vi "Example Callback - EdgeCount Callback.vi"(4 "EdgeCount":refnum<user-event>, 5 "Event Data":T1, 6 "Control Ref":refnum<k24>, 7 "Event Common Data":T2) -> ()   [LabVIEW 2013]
uses:
  C:/tf/play/labview/Tinkerforge.dll
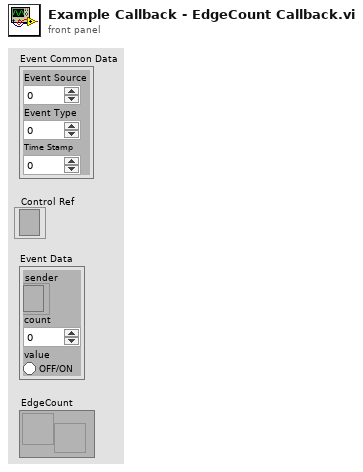
[diagram p1: front panel]
types:
  T1 = cluster{"sender":refnum<k24>, "count":i64, "value":bool}
  T2 = cluster{"Event Source":i32, "Event Type":u32, "Time Stamp":u32}
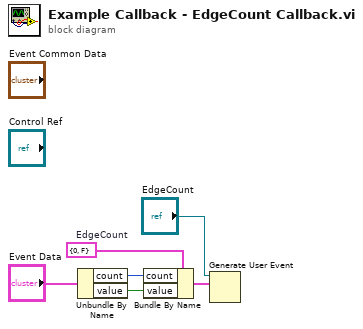
[diagram p0: block diagram]
diagram:
  w5 = cluster{"count":i64, "value":bool} {"count"=0, "value"=FALSE}  # EdgeCount
  n1 = Unbundle By Name("Event Data") -> ("count"=w3:i64, "value"=w4:bool)
  n2 = Bundle By Name(cluster=w5, "count"=w3, "value"=w4) -> (w2:cluster{"count":i64, "value":bool})
  n3 = Generate User Event(user event="EdgeCount", event data cluster=w2) -> ()  [unwired: 2 in, 2 out]
